vi "Cleanup.vi"(8 "error in (no error)":errorcluster, 11 "Config Manager in":refnum<class "Config Manager.lvclass">) -> (0 "error out":errorcluster)   [LabVIEW 2020, in "CDM-Config.lvlib" / "Config Manager.lvclass"]
doc: "Releases resources used to manage the Config. All elements owned by the config will be released as well and any further attempts to access the Config from other branches of its wire or any contained elements will fail.\n\nThis VI should be called for all Configs that are loaded or initialized except when a config has been merged into another config and automatically disposed."
uses:
  Config Manager.lvclass
  Config Manager.lvclass/Config Manager.ctl
  Config Element/Config Element.lvclass
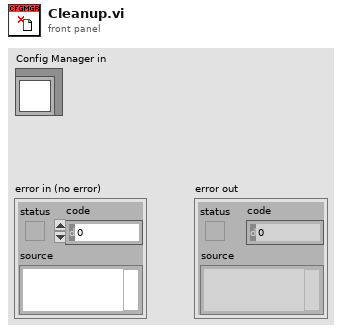
[diagram p1: front panel]
types:
  T1 = typedef "CDM-Config.lvlib/Config Manager.lvclass/Ref Data.ctl" = cluster{"Elements":refnum<class "Config Element.lvclass">[], "Hierarchy Map":map{string[], i32}, "Element Map":map{refnum<class "Config Element.lvclass">, i32}}
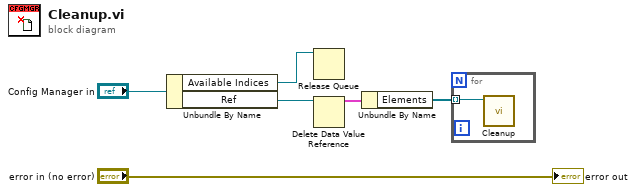
[diagram p0: block diagram]
diagram:
  n1 = Unbundle By Name("Config Manager in") -> ("Available Indices"=w1:refnum<queue>, "Ref"=w4:refnum<data-value>)
  n2 = Release Queue(queue=w1) -> ()  [unwired: 2 in, 3 out]
  n3 = Delete Data Value Reference(data value reference=w4) -> (data value=w3:T1)  [unwired: 1 in, 1 out]
  n4 = Unbundle By Name(w3) -> ("Elements"=w2:refnum<class "Config Element.lvclass">[])
  n5 = for {
    tunnel: w2 -> [w7] mode=indexing
    n6 = call "Cleanup.vi"("Config Element in"=w7) -> ()  [unwired: 10 in, 1 out]
  }
  "error out" <- "error in (no error)"
